vi "Start Logger.vi"(8 "error in (no error)":errorcluster, 11 "Monitor Controller in":refnum<class "Monitor Controller.lvclass">) -> (0 "error out":errorcluster, 2 "File Path":path, 3 "Monitor Controller out":refnum<class "Monitor Controller.lvclass">)   [LabVIEW 2018, in "Monitor Controller.lvclass"]
uses:
  Monitor Controller.lvclass
  C:/github/LabActor/Template Module/Template Module.lvclass
  C:/github/LabActor/Worker/Worker.lvclass
  C:/Program Files/National Instruments/LabVIEW 2018/vi.lib/ActorFramework/Actor/Actor.lvclass
  Template Module/Template Module.lvclass/Template Module.ctl
  Loggers/Logger/Logger.lvclass/Logger.ctl
  Worker/Worker.lvclass/Worker.ctl
  <vilib>/ActorFramework/Actor/Actor.lvclass/Actor.ctl
  LabActor Messages/Write Monitor File Msg/Write Monitor File Msg.lvclass/Write Monitor File Msg.ctl
  <vilib>/ActorFramework/Message Enqueuer/Message Enqueuer.lvclass/Message Enqueuer.ctl
  Update Monitor State Msg/Update Monitor State Msg.lvclass/Update Monitor State Msg.ctl
  Template Module/Read Logger.vi
  Loggers/Logger/Write Clean-up period.vi
  Template Module/Write Logger.vi
  Worker/Write Use buffered logger.vi
  <vilib>/ActorFramework/Message Enqueuer/Enqueue.vi
  LabActor Messages/Write Monitor File Msg/Write Monitor File Msg.lvclass
  C:/Program Files/National Instruments/LabVIEW 2018/vi.lib/ActorFramework/Message/Message.lvclass
  Update Monitor State Msg/Update Monitor State Msg.lvclass
  Read Monitor controller configuration.vi
  <vilib>/ActorFramework/Message Priority Queue/Priority Enqueue.vi
  Loggers/Logger/Logger.lvclass
  Process Controller/Process Controller.lvclass
  <vilib>/ActorFramework/Actor/Actor.lvclass
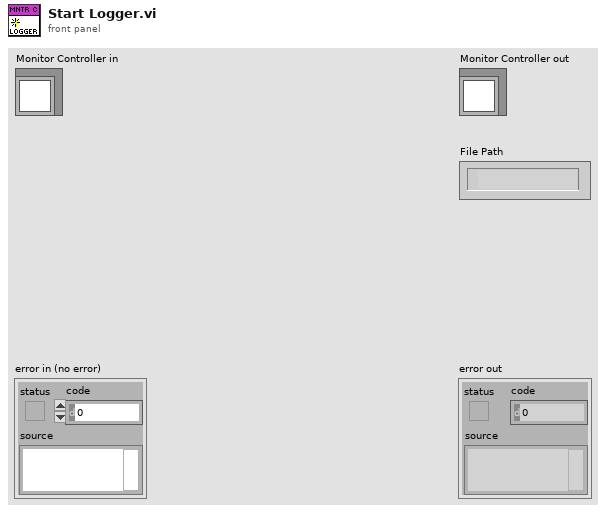
[diagram p1: front panel]
types:
  T1 = typedef "Monitor Controller Configuration.ctl" = cluster{"Update period":dbl, "Repeat times":i32, "Open plot":bool, "File defragment period":dbl, "Timestamp data points":bool, "Re-plot rate limit":dbl}
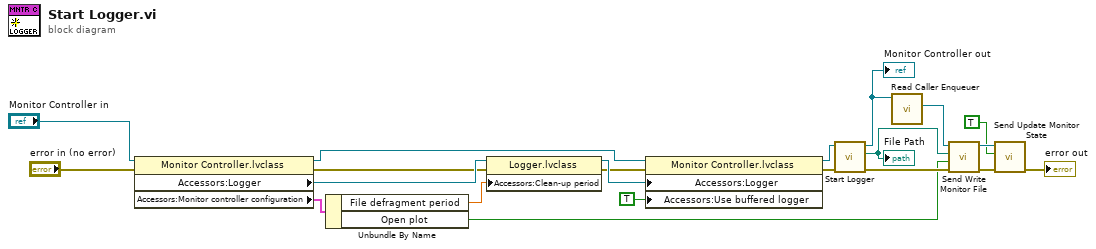
[diagram p0: block diagram]
diagram:
  n1 = property class="Monitor Controller.lvclass"(reference="Monitor Controller in", error in="error in (no error)") -> (reference out=w7:refnum<class "Monitor Controller.lvclass">, error out=w8:errorcluster, "Accessors:Logger"=w10:refnum<class "Logger.lvclass">, "Accessors:Monitor controller configuration"=w11:T1)
  n2 = Unbundle By Name(w11) -> ("File defragment period"=w9:dbl, "Open plot"=w1:bool)
  n3 = property class="Logger.lvclass"(reference=w10, error in=w8, "Accessors:Clean-up period"=w9) -> (reference out=w6:refnum<class "Logger.lvclass">, error out=w5:errorcluster)
  n4 = property class="Monitor Controller.lvclass"(reference=w7, error in=w5, "Accessors:Logger"=w6, "Accessors:Use buffered logger"=TRUE ("Use buffered logger")) -> (reference out=w3:refnum<class "Monitor Controller.lvclass">, error out=w4:errorcluster)
  n5 = call-parent "Start Logger.vi"("error in (no error)"=w4, "Measure Controller in"=w3) -> ("error out"=w17:errorcluster, "File Path"=w19:path, "Measure Controller out"=w18:refnum<class "Monitor Controller.lvclass">)  [unwired: 7 in]
  "Monitor Controller out" <- w18
  "File Path" <- w19
  n6 = call <vilib>:"Read Caller Enqueuer.vi"("Actor"=w18) -> ("Caller Enqueuer"=w20:refnum<class "Message Enqueuer.lvclass">)  [unwired: 10 in]
  n7 = call "Send Write Monitor File.vi"("error in (no error)"=w17, "Open plot"=w1, "Monitor File"=w19, "Message Enqueuer"=w20) -> ("error out"=w16:errorcluster, "Message Enqueuer out"=w15:refnum<class "Message Enqueuer.lvclass">)  [unwired: 6 in]
  n8 = call "Send Update Monitor State.vi"("error in (no error)"=w16, "Monitor Running"=TRUE, "Message Enqueuer"=w15) -> ("error out"=→"error out":errorcluster)  [unwired: 7 in, 1 out]
